vi "oa_Buffer Colormap.vi"(5 "plot type":T1(ring)=enum."Time-Frequency", 6 "number of spectra (40)":i32=40 min=1, 7 "reset? (F)":bool, 8 "error in":errorcluster, 11 "colormap in":T2={"value"=array1024x10[10240 elements], "x scale"={"offset"=0.0, "multiplier"=4.8828125}, "y scale"={"offset"=8.9, "multiplier"=0.1}, "attribute"=variant("NI_OAT_Plot_Type"=variant(enum16{"Frequency-Time", "Time-Frequency", "Order-Time", "Time-Order", "Frequency-RPM", "RPM-Frequency", "Order-RPM", "RPM-Order"} enum."Time-Frequency"), "NI_OAT_Speed_Profile"=variant(cluster{"time [s]":dbl[], "speed [rpm]":dbl[]} {"time [s]"=[8.89198317579559, 8.92846978699482, 8.966070912686485, 9.004895387154791, 9.04507100433862, 9.086749486770746, 9.13011327567989, 9.175385016398895, 9.22284117460173, 9.272832223229694, 9.32579662085929, 9.381810274589542, 9.440234081465459, 9.500000000000004, 9.560000000000002, 9.620000000000001, 9.680000000000001, 9.74, 9.800000000000004], "speed [rpm]"=[1663.7053584570283, 1615.2573158379785, 1565.2699992942808, 1513.5819780667632, 1460.0005299715128, 1404.292083502067, 1346.1685392608647, 1285.3173245721507, 1222.7107511996762, 1161.690452674099, 1107.0046394097117, 1063.1232664639783, 1031.877766676721, 1012.8074891903102, 1003.5236742900757, 1000.4181774161448, 1000.0000000000076, 999.9999999999936, 999.9999999999931]}))}) -> (0 "error out":errorcluster, 3 "colormap out":T2={"value"=array1024x90[92160 elements], "x scale"={"offset"=0.0, "multiplier"=0.1}, "y scale"={"offset"=0.0, "multiplier"=0.0}, "attribute"=variant})   [LabVIEW 2017]
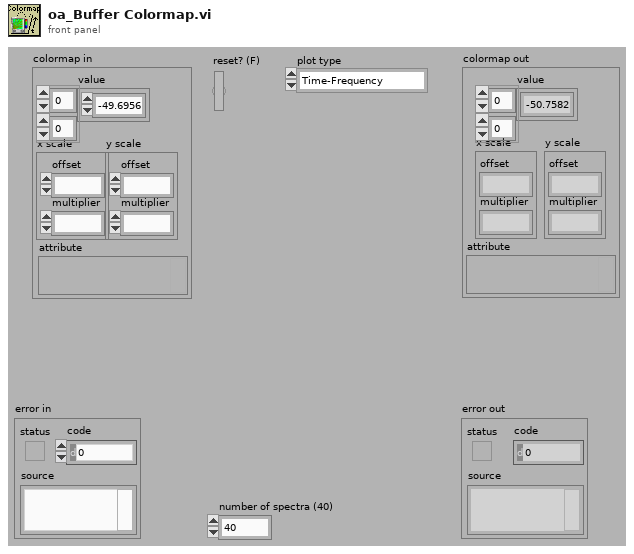
[diagram p1: front panel]
types:
  T1 = enum16{"Frequency-Time", "Time-Frequency", "Order-Time", "Time-Order", "Frequency-RPM", "RPM-Frequency", "Order-RPM", "RPM-Order"}
  T2 = cluster{"value":dbl[][], "x scale":cluster{"offset":dbl, "multiplier":dbl}, "y scale":cluster{"offset":dbl, "multiplier":dbl}, "attribute":variant}
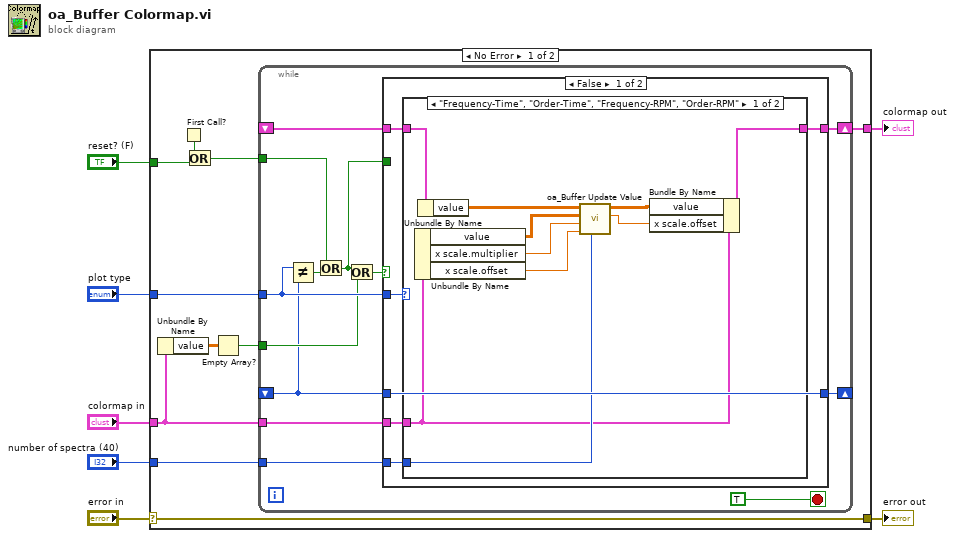
[diagram p0: block diagram]
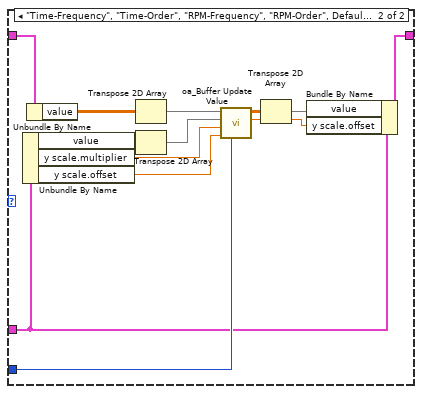
[diagram p2: hidden frame]
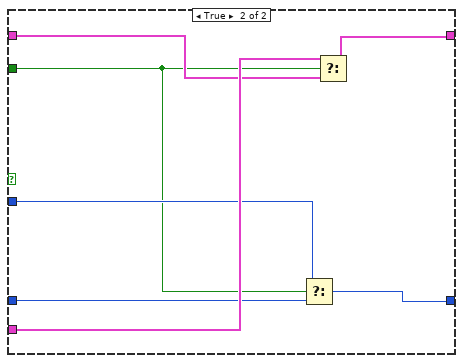
[diagram p3: hidden frame]
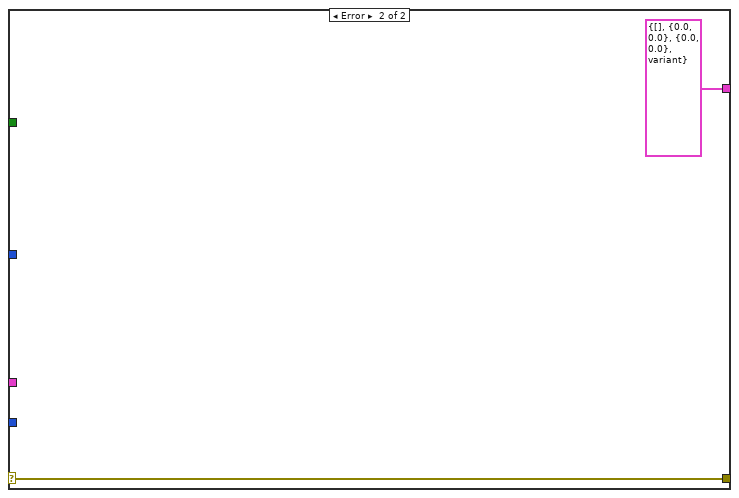
[diagram p4: hidden frame]
diagram:
  n1 = case shown="No Error" "error in" {
    selector: "error in" -> [w17 w68]
    tunnel: [w17 w68] -> w6
    tunnel: "colormap in" -> [w14 _]
    tunnel: "plot type" -> [w16 _]
    tunnel: "reset? (F)" -> [w12 _]
    tunnel: [w8 T2 {"value"=[], "x scale"={"offset"=0.0, "multiplier"=0.0}, "y scale"={"offset"=0.0, "multiplier"=0.0}, "attribute"=variant} ("colormap in")] -> w1
    tunnel: "number of spectra (40)" -> [w15 _]
    frame No Error {
      n2 = Unbundle By Name(w14) -> ("value"=w9:dbl[][])
      n3 = First Call?() -> (First Call?: T/F=w13:bool)
      n4 = Or(x=w13, y=w12) -> (x .or. y?=w11:bool)
      n5 = Empty Array?(array=w9) -> (empty?=w10:bool)
      n6 = while {
        tunnel: w16 -> [w28]
        tunnel: w14 -> [w24]
        shift-right: [w29] -> _
        shift-left: _ -> [w18]
        shift-right: [w23] -> w8
        shift-left: _ -> [w27]
        tunnel: w15 -> [w26]
        tunnel: w11 -> [w25]
        tunnel: w10 -> [w21]
        stop <- TRUE stop-if-true
        n7 = Not Equal?(x=w28, y=w18) -> (x != y?=w22:bool)
        n8 = Or(x=w25, y=w22) -> (x .or. y?=w19:bool)
        n9 = Or(x=w19, y=w21) -> (x .or. y?=w20:bool)
        n10 = case shown="False" w20 {
          tunnel: w28 -> [w32 w63]
          tunnel: w26 -> [w36 _]
          tunnel: w24 -> [w35 w66]
          tunnel: w27 -> [w34 w65]
          tunnel: [w33 w64] -> w23
          tunnel: [w31 w61] -> w29
          tunnel: w19 -> [_ w60]
          tunnel: w18 -> [w31 w62]
          frame False {
            n11 = case shown="\"Frequency-Time\", \"Order-Time\", \"Frequency-RPM\", \"Order-RPM\"" w32 {
              tunnel: w35 -> [w38 w48]
              tunnel: w34 -> [w46 w56]
              tunnel: w36 -> [w41 w51]
              tunnel: [w37 w47] -> w33
              frame "Frequency-Time", "Order-Time", "Frequency-RPM", "Order-RPM" {
                n12 = Unbundle By Name(w38) -> ("value"=w44:dbl[][], "x scale.multiplier"=w43:dbl, "x scale.offset"=w42:dbl)
                n13 = Unbundle By Name(w46) -> ("value"=w45:dbl[][])
                n14 = call <vilib>:"oa_Buffer Update Value.vi"("number of spectra (40)"=w41, "current offset"=w42, "current multiplier"=w43, "current value"=w44, "previous value"=w45) -> ("Offset"=w39:dbl, "value"=w40:dbl[][])  [unwired: 4 in, 1 out]
                n15 = Bundle By Name(cluster=w38, "value"=w40, "x scale.offset"=w39) -> (w37:T2)
              }
              frame "Time-Frequency", "Time-Order", "RPM-Frequency", "RPM-Order", Default {
                n16 = Unbundle By Name(w48) -> ("value"=w58:dbl[][], "y scale.multiplier"=w53:dbl, "y scale.offset"=w52:dbl)
                n17 = Unbundle By Name(w56) -> ("value"=w59:dbl[][])
                n18 = Transpose 2D Array(2D array=w59) -> (transposed array=w55:dbl[][])
                n19 = Transpose 2D Array(2D array=w58) -> (transposed array=w54:dbl[][])
                n20 = call <vilib>:"oa_Buffer Update Value.vi"("number of spectra (40)"=w51, "current offset"=w52, "current multiplier"=w53, "current value"=w54, "previous value"=w55) -> ("Offset"=w49:dbl, "value"=w50:dbl[][])  [unwired: 4 in, 1 out]
                n21 = Transpose 2D Array(2D array=w50) -> (transposed array=w57:dbl[][])
                n22 = Bundle By Name(cluster=w48, "value"=w57, "y scale.offset"=w49) -> (w47:T2)
              }
            }
          }
          frame True {
            n23 = Select(t=w63, s=w60, f=w62) -> (s? t:f=w61:T1)
            n24 = Select(t=w66, s=w60, f=w65) -> (s? t:f=w64:T2)
          }
        }
      }
    }
    frame Error {
    }
  }
  "colormap out" <- w1
  "error out" <- w6
